vi "CU_addTestTrials.vi"(8 "error in (no error)":errorcluster, 11 "ClassifierClass in":refnum<class "ClassifierClass.lvclass">) -> (0 "error out":errorcluster, 1 "FeatureVectorLength":i32, 2 "Array of Test Trials out":T1[](array[typedef]), 3 "ClassifierClass out":refnum<class "ClassifierClass.lvclass">)   [LabVIEW 2016, in "Classifier.lvlib" / "ClassifierClass.lvclass"]
uses:
  ClassifierClass.lvclass
  _XML_EEG_Features/XML_FF_Trial.ctl
  ClassifierClass.lvclass/ClassifierClass.ctl
  <vilib>/xml/Close Reference(Node).vi
  _XML_EEG_Features/XML_EEG_Features.lvlib
  <vilib>/xml/NI_XML.lvlib
panel:
  # "This VI is a part of BCI Design library, http://www.ru-bci.org \nCopyright © 2020, Sotnikov Peter, All rights reserved. License: GNU GPLv3"
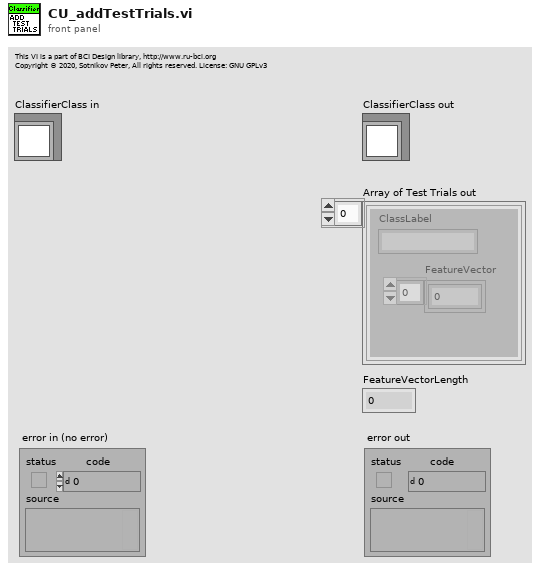
[diagram p1: front panel]
types:
  T1 = typedef "XML_EEG_Features.lvlib/XML_FF_Trial.ctl" = cluster{"ClassLabel":string, "FeatureVector":dbl[]}
  T2 = typedef "XML_EEG_Features.lvlib/XML_FF_Header.ctl" = cluster{"NumberOfTrials":i32, "NumberOfClasses":i32, "FeatureVectorLength":i32, "FeatureExtractionMethod":string}
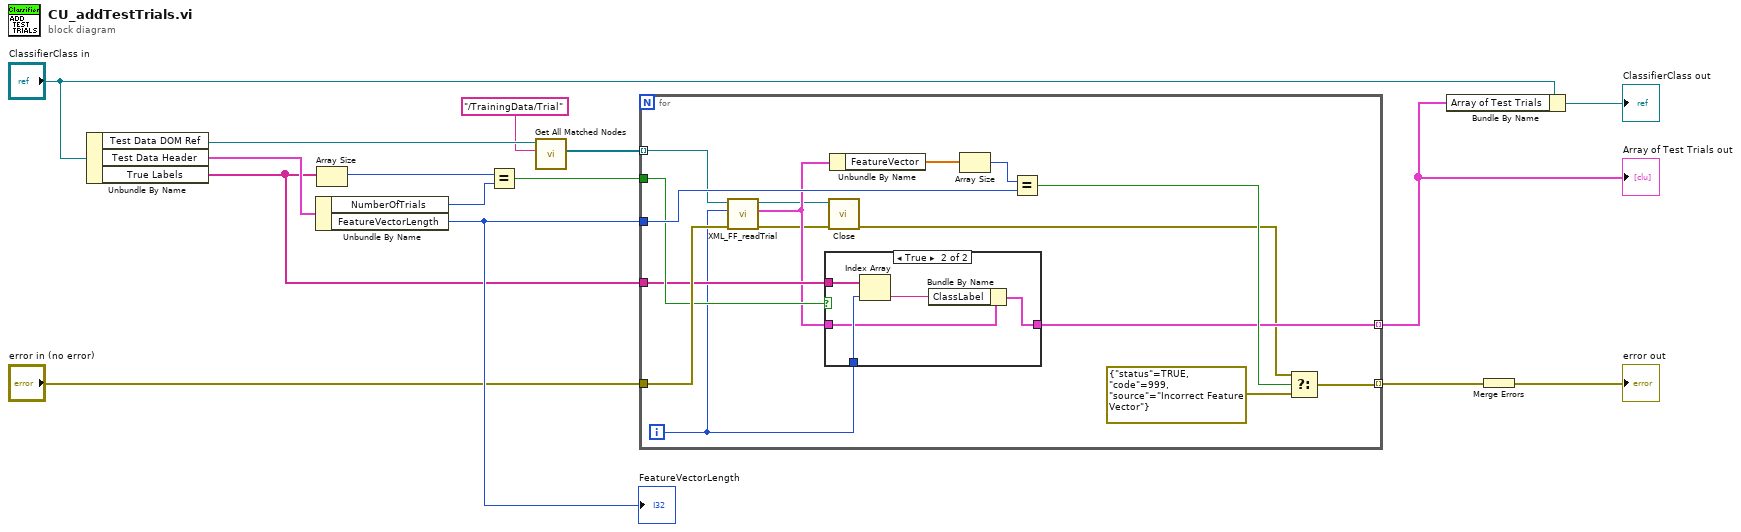
[diagram p0: block diagram]
diagram:
  n1 = Unbundle By Name("ClassifierClass in") -> ("Test Data DOM Ref"=w3:refnum<k20>, "Test Data Header"=w11:T2, "True Labels"=w4:string[])
  n2 = Unbundle By Name(w11) -> ("NumberOfTrials"=w6:i32, "FeatureVectorLength"=w15:i32)
  "FeatureVectorLength" <- w15
  n3 = Array Size(array=w4) -> (size(s)=w7:i32)
  n4 = Equal?(x=w7, y=w6) -> (x = y?=w5:bool)
  n5 = call <vilib>:"Get All Matched Nodes.vi"("XPath expression"="/TrainingData/Trial", "node in"=w3) -> ("node result array"=w2:refnum<k20>[])  [unwired: 7 in, 2 out]
  n6 = for {
    tunnel: "error in (no error)" -> [w31]
    tunnel: w15 -> [w29]
    tunnel: [w27] -> w13 mode=indexing
    tunnel: [w19] -> w8 mode=indexing
    tunnel: w5 -> [w23]
    tunnel: w4 -> [w22]
    tunnel: w2 -> [w24] mode=indexing
    i -> [w21]
    n7 = call "XML_FF_readTrial.vi"("error in (no error)"=w31, "Trial Number"=w21, "DOM document in"=w24) -> ("error out"=w18:errorcluster, "Trial out"=w20:T1, "DOM document out"=w17:refnum<k20>)  [unwired: 6 in]
    n8 = case shown="True" w23 {
      tunnel: w22 -> [_ w37]
      tunnel: w21 -> [_ w36]
      tunnel: w20 -> [w32 w34]
      tunnel: [w32 w33] -> w19
      frame False {
      }
      frame True {
        n9 = Index Array(array=w37, index=w36) -> (element=w35:string)
        n10 = Bundle By Name(cluster=w34, "ClassLabel"=w35) -> (w33:T1)
      }
    }
    n11 = call-poly <vilib>:"Close.vi"("error in (no error)"=w18, "node"=w17) -> ("error out"=w16:errorcluster)  [unwired: 7 in]
    n12 = Unbundle By Name(w20) -> ("FeatureVector"=w28:dbl[])
    n13 = Array Size(array=w28) -> (size(s)=w30:i32)
    n14 = Equal?(x=w30, y=w29) -> (x = y?=w26:bool)
    n15 = Select(t=w16, s=w26, f=errorcluster {"status"=TRUE, "code"=999, "source"="Incorrect Feature Vector"} ("error out")) -> (s? t:f=w27:errorcluster)
  }
  "Array of Test Trials out" <- w8
  n16 = Bundle By Name(cluster="ClassifierClass in", "Array of Test Trials"=w8) -> (→"ClassifierClass out":refnum<class "ClassifierClass.lvclass">)
  n17 = Merge Errors(w13) -> (→"error out":errorcluster)
